vi "Populate Tests.vi"(8 "error in (no error)":errorcluster, 10 "Test Finder in":refnum<class "Test Finder.lvclass">, 11 "Test Tree In":refnum<class "Test Result Tree.lvclass">) -> (0 "error out":errorcluster, 2 "Test Case Finder Out":refnum<class "Test Finder.lvclass">, 3 "Test Tree Out":refnum<class "Test Result Tree.lvclass">)   [LabVIEW 2020, in "Test Result Tree.lvclass"]
uses:
  Test Result Tree/Test Result Tree.lvclass
  Test Finder/Test Finder.lvclass
  C:/Users/anton/Documents/GitHub/LUnit/source/Framework/Helper Classes/Test Tree/Test Tree.lvclass
  Test Tree.lvclass/Test Tree.ctl
  <vilib>/Utility/miscctls.llb/LVMapReplaceAction.ctl
  Test Tree.lvclass
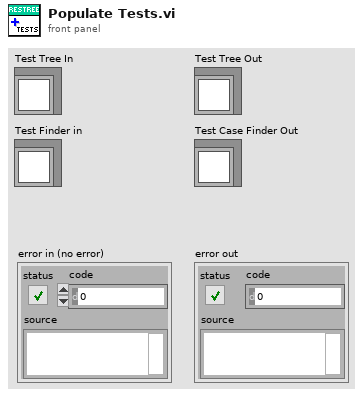
[diagram p1: front panel]
types:
  T1 = map{string, cluster{"Left Cell String":string, "Child Text":string[], "Item Indent":i32, "Child Only?":bool, "Glyph Index":i32}}
  T2 = typedef "LVMapReplaceAction.ctl" = enum32{"Modify Entry only if found", "Add or Modify Entry", "Delete Entry"}
  T3 = cluster{"Left Cell String":string, "Child Text":string[], "Item Indent":i32, "Child Only?":bool, "Glyph Index":i32}
  T4 = cluster{"Method Name":string, "Fully Qualified Name":string}[]
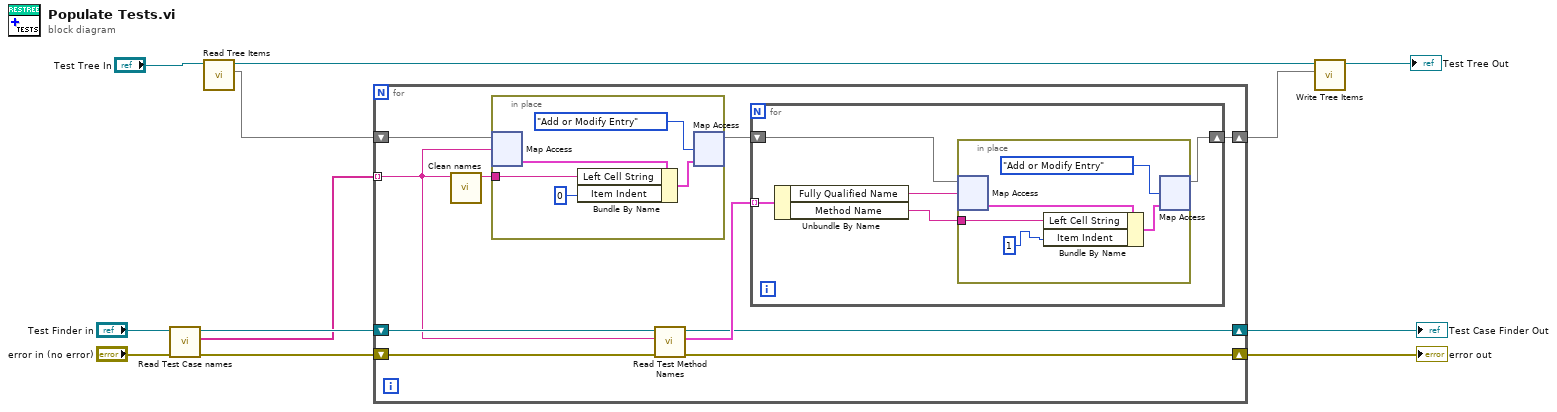
[diagram p0: block diagram]
diagram:
  n1 = call "Read Test Case names.vi"("error in (no error)"="error in (no error)", "Test Case Finder In"="Test Finder in") -> ("error out"=w8:errorcluster, "Test Cases"=w10:string[], "Test Case Finder Out"=w12:refnum<class "Test Finder.lvclass">)  [unwired: 7 in]
  n2 = call "Read Tree Items.vi"("Test Tree In"="Test Tree In") -> ("Tree Items"=w1:T1, "Test Tree Out"=w2:refnum<class "Test Result Tree.lvclass">)  [unwired: 9 in]
  n3 = for {
    tunnel: w10 -> [w14] mode=indexing
    shift-right: [w18] -> w6
    shift-left: w8 -> [w19]
    shift-right: [w20] -> w9
    shift-left: w12 -> [w21]
    shift-right: [w17] -> w4
    shift-left: w1 -> [w16]
    n4 = call "Clean names.vi"("Name with extension"=w14) -> ("Name without extension"=w13:string)  [unwired: 10 in]
    n5 = in-place {
      in-place-border: w13 -> [w25]
      n6 = in-place-map #1(w16, w14) -> (w26:T3)  [unwired: 1 in, 1 out]
      n7 = Bundle By Name(cluster=w26, "Left Cell String"=w25, "Item Indent"=0 ("New Item Indentation")) -> (w24:T3)
      n8 = in-place-map #1(w24, LVMapReplaceAction."Add or Modify Entry" ("action")) -> (w15:T1)  [unwired: 2 out]
    }
    n9 = call "Read Test Method Names.vi"("error in (no error)"=w19, "Test Case"=w14, "Test Case Finder In"=w21) -> ("error out"=w18:errorcluster, "Names"=w22:T4, "Test Case Finder Out"=w20:refnum<class "Test Finder.lvclass">)  [unwired: 6 in]
    n10 = for {
      tunnel: w22 -> [w32] mode=indexing
      shift-right: [w28] -> w17
      shift-left: w15 -> [w31]
      n11 = Unbundle By Name(w32) -> ("Fully Qualified Name"=w30:string, "Method Name"=w29:string)
      n12 = in-place {
        in-place-border: w29 -> [w36]
        n13 = in-place-map #2(w31, w30) -> (w37:T3)  [unwired: 1 in, 1 out]
        n14 = Bundle By Name(cluster=w37, "Left Cell String"=w36, "Item Indent"=1 ("New Item Indentation")) -> (w35:T3)
        n15 = in-place-map #2(w35, LVMapReplaceAction."Add or Modify Entry" ("action")) -> (w28:T1)  [unwired: 2 out]
      }
    }
  }
  "error out" <- w6
  "Test Case Finder Out" <- w9
  n16 = call "Write Tree Items.vi"("Tree Items"=w4, "Test Tree In"=w2) -> ("Test Tree Out"=→"Test Tree Out":refnum<class "Test Result Tree.lvclass">)  [unwired: 9 in]
